vi "Read DAQ FIFO.vi"(7 "Channel Index":i32, 8 "error in (no error)":errorcluster, 9 "Timeout (ms)":i32, 10 "Data In":T1[](array[typedef]), 11 "CIFCorePlugin in":refnum<class "CIFCorePlugin.lvclass">) -> (0 "error out":errorcluster, 1 "timed out?":bool, 2 "Data Out":T1[](array[typedef]), 3 "CIFCorePlugin out":refnum<class "CIFCorePlugin.lvclass">, 4 "Header":T2)   [LabVIEW 2021, in "CIFCorePlugin.lvclass"]
uses:
  CIFCorePlugin.lvclass
  <vilib>/CIF Foundation/CIF Channels Core/CIFChannels/CIFChannels.lvclass
  <vilib>/CIF Foundation/CIF Channels Core/ChannelCommon/typedef/FIFO Header.ctl
  <vilib>/CIF Foundation/CIF Channels Core/ChannelCommon/ChannelCommon.lvlib
  <vilib>/CIF Foundation/CIF Channels Core/ChannelCommon/typedef/Datatype Waveform.ctl
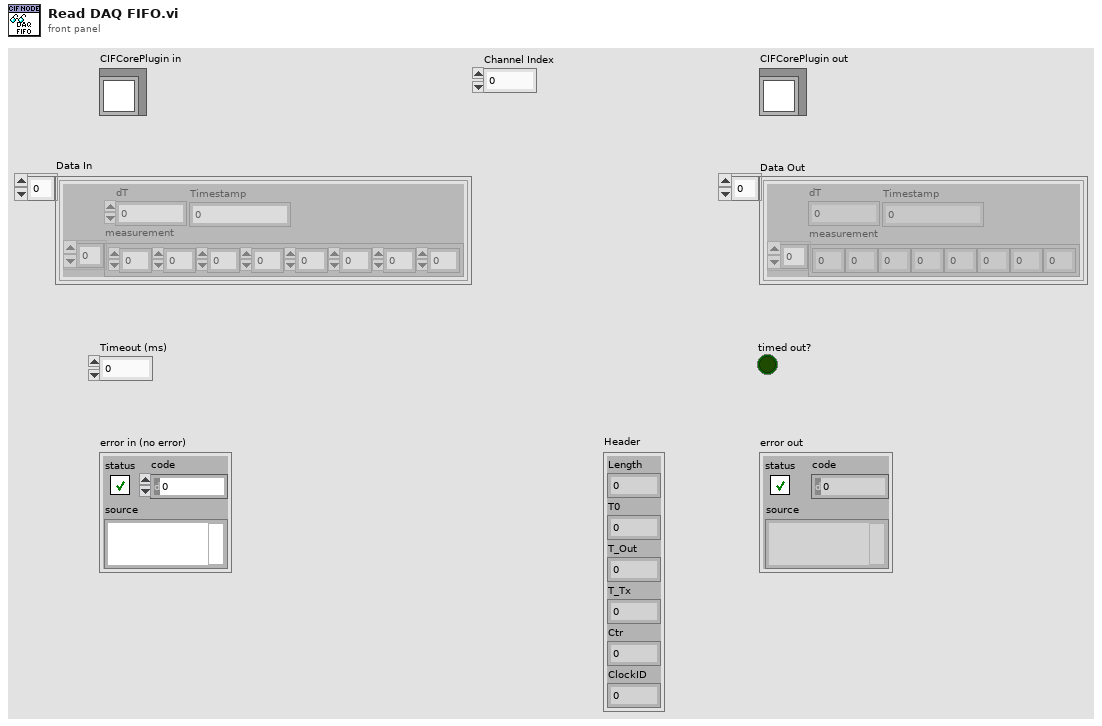
[diagram p1: front panel]
types:
  T1 = typedef "ChannelCommon.lvlib/Datatype Waveform.ctl" = cluster{"measurement":dbl[], "dT":dbl, "Timestamp":i64}
  T2 = typedef "ChannelCommon.lvlib/FIFO Header.ctl" = cluster{"Length":u64, "T0":i64, "T_Out":i64, "T_Tx":i64, "Ctr":u64, "ClockID":u8}
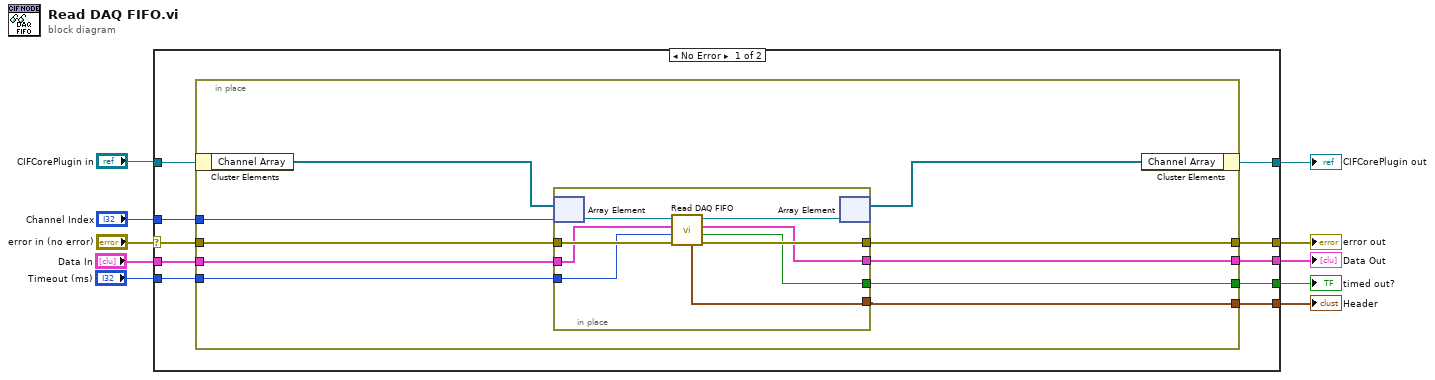
[diagram p0: block diagram]
diagram:
  n1 = case shown="No Error" "error in (no error)" {
    selector: "error in (no error)" -> [w20 w41]
    tunnel: [w19 w41] -> w8
    tunnel: [w16 w40] -> w9
    tunnel: "CIFCorePlugin in" -> [w17 w40]
    tunnel: [w18 _] -> w1
    tunnel: "Channel Index" -> [w15 _]
    tunnel: "Timeout (ms)" -> [w14 _]
    tunnel: [w13 _] -> w4
    tunnel: [w12 _] -> w3
    tunnel: "Data In" -> [w11 _]
    frame No Error {
      n2 = in-place {
        in-place-border: w20 -> [w21]
        in-place-border: [w22] -> w19
        in-place-border: [w30] -> w18
        in-place-border: w15 -> [w29]
        in-place-border: w14 -> [w28]
        in-place-border: [w27] -> w13
        in-place-border: [w26] -> w12
        in-place-border: w11 -> [w25]
        n3 = in-place-cluster #1(w17) -> ("Channel Array"=w24:refnum<class "CIFChannels.lvclass">[])
        n4 = in-place {
          in-place-border: w21 -> [w39]
          in-place-border: [w38] -> w22
          in-place-border: [w35] -> w30
          in-place-border: w28 -> [w34]
          in-place-border: [w33] -> w27
          in-place-border: [w32] -> w26
          in-place-border: w25 -> [w31]
          n5 = in-place-array #2(w24, w29) -> (w37:refnum<class "CIFChannels.lvclass">)
          n6 = call-dynamic "Read DAQ FIFO.vi"("error in (no error)"=w39, "Timeout (ms)"=w34, "Data In"=w31, "CIFChannels in"=w37) -> ("error out"=w38:errorcluster, "timed out?"=w33:bool, "Data Out"=w35:T1[], "CIFChannels out"=w36:refnum<class "CIFChannels.lvclass">, "Header"=w32:T2)  [unwired: 3 in]
          n7 = in-place-array #2(w36) -> (w23:refnum<class "CIFChannels.lvclass">[])  [unwired: 1 out]
        }
        n8 = in-place-cluster #1("Channel Array"=w23) -> (w16:refnum<class "CIFCorePlugin.lvclass">)
      }
    }
    frame Error {
    }
  }
  "error out" <- w8
  "CIFCorePlugin out" <- w9
  "timed out?" <- w4
  "Header" <- w3
  "Data Out" <- w1
